vi "Create Resource Name.vi"(8 "error in (no error)":errorcluster, 9 "Filter Type":T1, 10 "Filter List":string[](array[string]), 11 "System Hardware Ref":refnum<k20>) -> (0 "error out":errorcluster, 1 "Alias":string[](array[string]), 2 "Use":bool, 3 "Name and Alias":string[](array[string]))   [LabVIEW 2019, in "NIVS Hardware Discovery.lvlib"]
uses:
  NIVS Hardware Discovery.lvlib
  Types/Filter Type.ctl
  <resource>/objmgr/nicontrollersysapi.rc
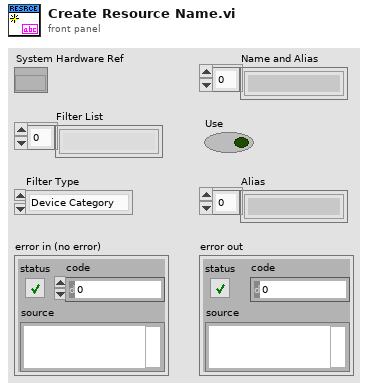
[diagram p1: front panel]
types:
  T1 = typedef "NIVS Hardware Discovery.lvlib/Filter Type.ctl" = enum16{"Device Category", "Product Name", "Ethernet", "XNET", "VISA", "FPGA", "EtherCAT Master", "DAQmx", "GPIB", "Serial"}
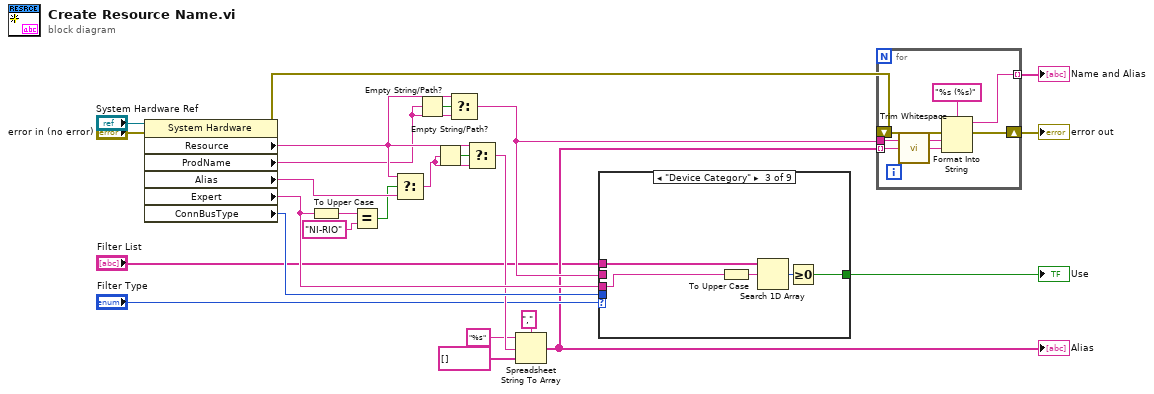
[diagram p0: block diagram]
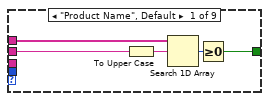
[diagram p2: hidden frame]
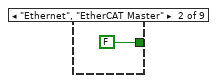
[diagram p3: hidden frame]
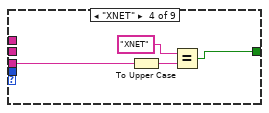
[diagram p4: hidden frame]
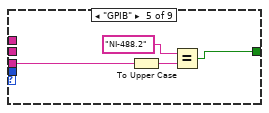
[diagram p5: hidden frame]
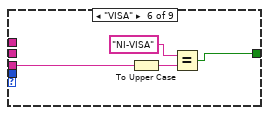
[diagram p6: hidden frame]
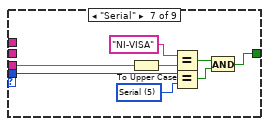
[diagram p7: hidden frame]
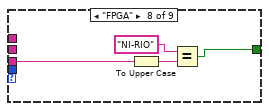
[diagram p8: hidden frame]
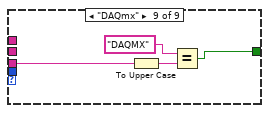
[diagram p9: hidden frame]
diagram:
  n1 = property class="System Hardware"(reference="System Hardware Ref", error in="error in (no error)") -> (error out=w25:errorcluster, "Resource"=w21:string, "ProdName"=w14:string, "Alias"=w23:string, "Expert"=w19:string, "ConnBusType"=w24:u32)  [unwired: 1 out]
  n2 = To Upper Case(1:w19) -> (0:w17:string)
  n3 = Equal?(x=w17, y="NI-RIO" ("x")) -> (x = y?=w20:bool)
  n4 = Select(t=w21, s=w20, f=w23) -> (s? t:f=w22:string)
  n5 = Empty String/Path?(string/path=w14) -> (empty?=w10:bool)
  n6 = Empty String/Path?(string/path=w22) -> (empty?=w11:bool)
  n7 = Select(t=w21, s=w10, f=w14) -> (s? t:f=w12:string)
  n8 = Select(t=w21, s=w11, f=w22) -> (s? t:f=w13:string)
  n9 = Spreadsheet String To Array(delimiter (Tab)=",", format string="%s", spreadsheet string=w13, array type (2D Dbl)=string[] []) -> (array=w8:string[])
  "Alias" <- w8
  n10 = case shown="\"Device Category\"" "Filter Type" {
    tunnel: "Filter List" -> [w30 _ w36 _ _ _ _ _ _]
    tunnel: w12 -> [w29 _ _ _ _ _ _ _ _]
    tunnel: [w27 FALSE w34 w38 w42 w46 w50 w58 w62] -> w4
    tunnel: w19 -> [_ _ w33 w40 w44 w48 w56 w60 w64]
    tunnel: w24 -> [_ _ _ _ _ _ w49 _ _]
    frame "Product Name", Default {
      n11 = To Upper Case(1:w29) -> (0:w26:string)
      n12 = Search 1D Array(1D array=w30, element=w26) -> (index of element=w28:i32)  [unwired: 1 in]
      n13 = Greater Or Equal To 0?(x=w28) -> (x >= 0?=w27:bool)
    }
    frame "Ethernet", "EtherCAT Master" {
    }
    frame "Device Category" {
      n14 = To Upper Case(1:w33) -> (0:w32:string)
      n15 = Search 1D Array(1D array=w36, element=w32) -> (index of element=w35:i32)  [unwired: 1 in]
      n16 = Greater Or Equal To 0?(x=w35) -> (x >= 0?=w34:bool)
    }
    frame "XNET" {
      n17 = To Upper Case(1:w40) -> (0:w39:string)
      n18 = Equal?(x="XNET", y=w39) -> (x = y?=w38:bool)
    }
    frame "GPIB" {
      n19 = To Upper Case(1:w44) -> (0:w43:string)
      n20 = Equal?(x="NI-488.2", y=w43) -> (x = y?=w42:bool)
    }
    frame "VISA" {
      n21 = To Upper Case(1:w48) -> (0:w47:string)
      n22 = Equal?(x="NI-VISA", y=w47) -> (x = y?=w46:bool)
    }
    frame "Serial" {
      w53 = u32 5 items=["BuiltIn/System", "PXI/PCI", "USB", "GPIB", "VXI", "Serial", "TCP/IP", "cRIO", "SCXI", "cDAQ", "SwitchBlock", "SCC", "FireWire", "Accessory", "CAN", "SwitchBlock Device"] ("Devices & Chassis:Connects To Bus Type")
      n23 = To Upper Case(1:w56) -> (0:w55:string)
      n24 = Equal?(x="NI-VISA", y=w55) -> (x = y?=w51:bool)
      n25 = Equal?(x=w49, y=w53) -> (x = y?=w52:bool)
      n26 = And(x=w51, y=w52) -> (x .and. y?=w50:bool)
    }
    frame "FPGA" {
      n27 = To Upper Case(1:w60) -> (0:w59:string)
      n28 = Equal?(x="NI-RIO", y=w59) -> (x = y?=w58:bool)
    }
    frame "DAQmx" {
      n29 = To Upper Case(1:w64) -> (0:w63:string)
      n30 = Equal?(x="DAQMX" ("Display"), y=w63) -> (x = y?=w62:bool)
    }
  }
  "Use" <- w4
  n31 = for {
    tunnel: w12 -> [w68]
    tunnel: w8 -> [w66] mode=indexing
    shift-right: [w69] -> w2
    shift-left: w25 -> [w70]
    tunnel: [w71] -> w1 mode=indexing
    n32 = call <vilib>:"Trim Whitespace.vi"("string"=w66) -> ("trimmed string"=w67:string)  [unwired: 1 in]
    n33 = Format Into String(format string="%s (%s)", error in=w70, w68, w67) -> (resulting string=w71:string, error out=w69:errorcluster)  [unwired: 1 in]
  }
  "error out" <- w2
  "Name and Alias" <- w1
